vi "element to byte index.vi"(7 "big endian?":bool, 9 "element number":i32, 10 "data type":T1, 11 "assembly size (bytes)":u32) -> (2 "subindex":i32, 3 "byte index":i32)   [LabVIEW 2013, in "EthernetIP Channel.lvclass"]
uses:
  EthernetIP Channel.lvclass
  <vilib>/NI/Tag Bus/tag/Data Type.ctl
  <vilib>/NI/Tag Bus/tag/tag descriptor.lvclass
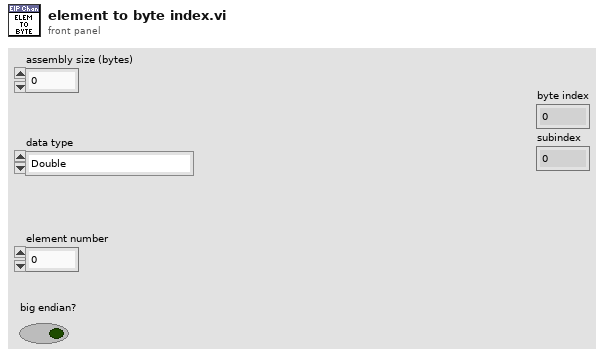
[diagram p1: front panel]
types:
  T1 = typedef "tag bus.lvlib/tag descriptor.lvclass/Data Type.ctl" = enum16{"Double", "Single", "I64", "I32", "I16", "I8", "U64", "U32", "U16", "U8", "Boolean", "String", "Array of Double", "Array of Single", "Array of I64", "Array of I32", "Array of I16", "Array of I8", "Array of U64", "Array of U32", "Array of U16", "Array of U8", "Array of Boolean", "Array of String"}
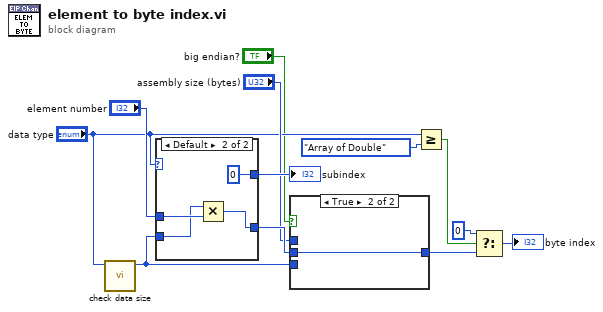
[diagram p0: block diagram]
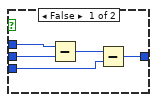
[diagram p2: hidden frame]
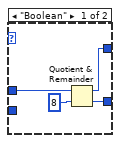
[diagram p3: hidden frame]
diagram:
  n1 = call "check data size.vi"("data type"="data type") -> ("bytes"=w9:i32)  [unwired: 10 in]
  n2 = case shown="Default" "data type" {
    tunnel: [w13 0 ("subindex 2")] -> w12
    tunnel: "element number" -> [w16 w19]
    tunnel: [w14 w18] -> w10
    tunnel: w9 -> [_ w17]
    frame "Boolean" {
      n3 = Quotient & Remainder(x=w16, y=8) -> (x-y*floor(x/y)=w13:i32, floor(x/y)=w14:i32)
    }
    frame Default {
      n4 = Multiply(x=w17, y=w19) -> (x*y=w18:i32)
    }
  }
  "subindex" <- w12
  n5 = case shown="True" "big endian?" {
    tunnel: [w21 w26] -> w3
    tunnel: w10 -> [w24 w26]
    tunnel: w9 -> [w23 _]
    tunnel: "assembly size (bytes)" -> [w25 _]
    frame False {
      n6 = Subtract(x=w25, y=w24) -> (x-y=w22:u32)
      n7 = Subtract(x=w22, y=w23) -> (x-y=w21:u32)
    }
    frame True {
    }
  }
  n8 = Greater Or Equal?(x="data type", y=Data_Type."Array of Double" ("x")) -> (x >= y?=w4:bool)
  n9 = Select(t=u32 0, s=w4, f=w3) -> (s? t:f=→"byte index":u32)
